vi "Initialize Product.vi"(8 "error in (no error)":errorcluster, 11 "Productos in":refnum<class "Productos.lvclass">) -> (0 "error out":errorcluster, 3 "Productos out":refnum<class "Productos.lvclass">)   [LabVIEW 2020, in "Productos.lvlib" / "Productos.lvclass"]
uses:
  Productos.lvclass
  Productos.lvclass/Productos.ctl
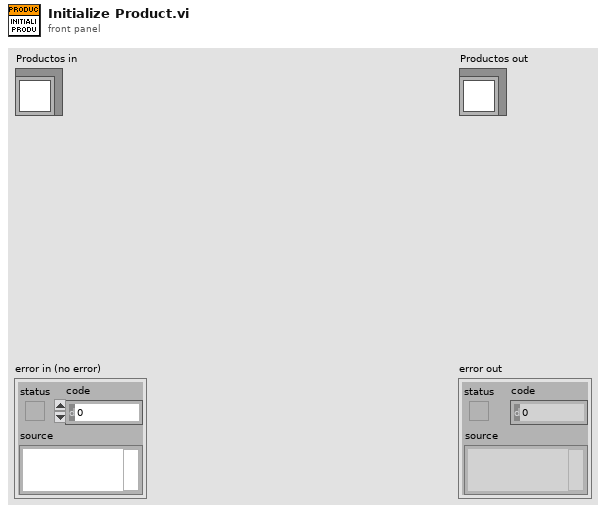
[diagram p1: front panel]
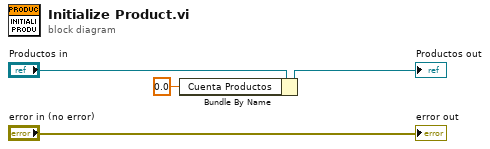
[diagram p0: block diagram]
diagram:
  n1 = Bundle By Name(cluster="Productos in", "Cuenta Productos"=0.0) -> (→"Productos out":refnum<class "Productos.lvclass">)
  "error out" <- "error in (no error)"
